vi "Cache.FindToExport.vi"(7 "Idx":i32, 8 "error in (no error)":errorcluster, 11 "Data in":T7) -> (0 "error out":errorcluster, 1 "ProductComponent":T1[](array[typedef]), 2 "Results":T2[](array[typedef]), 3 "Data out":T7)   [LabVIEW 2016]
uses:
  Cache.Data.ctl
  Cache.Data.Status.ctl
  Cache.Data.Sets.ctl
  Cache.TestSteps.Fglb.ResultData.ctl
  Database/ProdaNG/Controls/ProdaNG.ProcessResult.ctl
  Database/ProdaNG/Controls/ProdaNG.ProcessStepResult.ctl
  Database/ProdaNG/Controls/ProdaNG.TestStepResult.ctl
  Database/ProdaNG/Controls/ProdaNG.TestValueResult.ctl
  Database/ProdaNG/Controls/ProdaNG.ProductComponent.ctl
  Global/ApplicationGlobal.vi
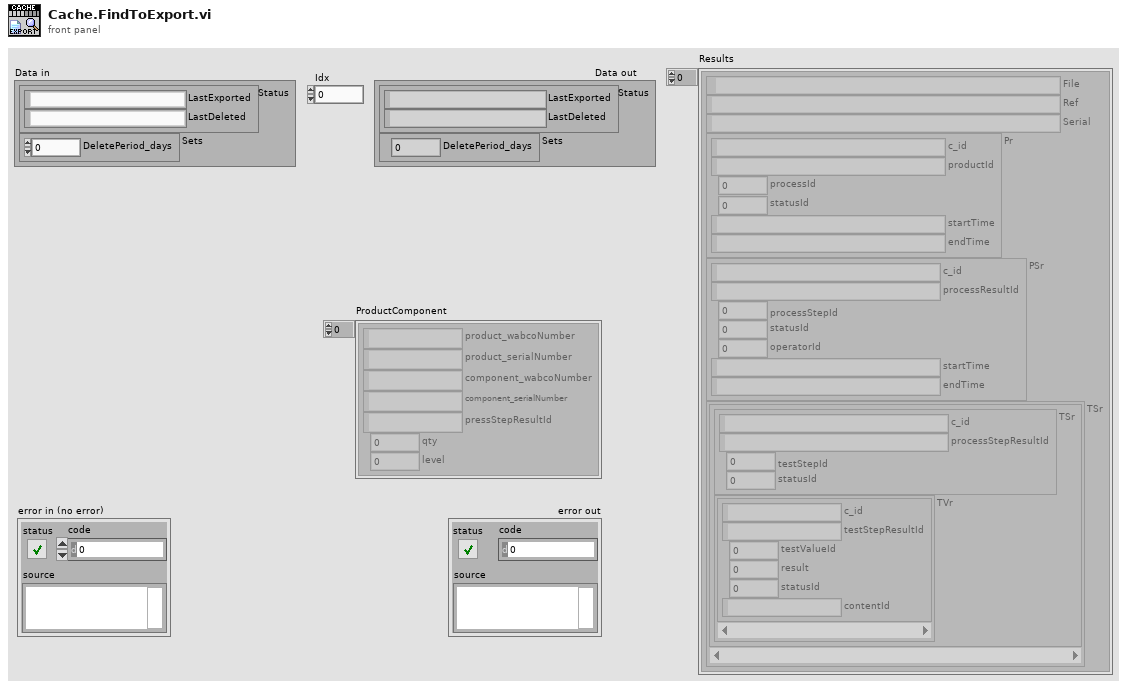
[diagram p1: front panel]
types:
  T1 = typedef "ProdaNG.ProductComponent.ctl" = cluster{"product_wabcoNumber":string, "product_serialNumber":string, "component_wabcoNumber":string, "component_serialNumber":string, "pressStepResultId":string, "qty":i32, "level":i32}
  T2 = typedef "Cache.TestSteps.Fglb.ResultData.ctl" = cluster{"File":path, "Ref":string, "Serial":string, "Pr":T3, "PSr":T4, "TSr":cluster{"TSr":T5, "TVr":T6[]}[]}
  T3 = typedef "ProdaNG.ProcessResult.ctl" = cluster{"c_id":string, "productId":string, "processId":i32, "statusId":i32, "startTime":string, "endTime":string}
  T4 = typedef "ProdaNG.ProcessStepResult.ctl" = cluster{"c_id":string, "processResultId":string, "processStepId":i32, "statusId":i32, "operatorId":i32, "startTime":string, "endTime":string}
  T5 = typedef "ProdaNG.TestStepResult.ctl" = cluster{"c_id":string, "processStepResultId":string, "testStepId":i32, "statusId":i32}
  T6 = typedef "ProdaNG.TestValueResult.ctl" = cluster{"c_id":string, "testStepResultId":string, "testValueId":i32, "result":dbl, "statusId":i32, "contentId":string}
  T7 = typedef "Cache.Data.ctl" = cluster{"Status":T8, "Sets":T9}
  T8 = typedef "Cache.Data.Status.ctl" = cluster{"LastExported":string, "LastDeleted":string}
  T9 = typedef "Cache.Data.Sets.ctl" = cluster{"DeletePeriod_days":dbl}
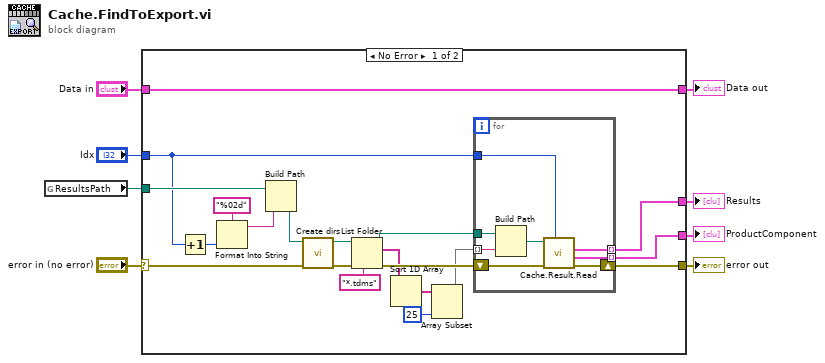
[diagram p0: block diagram]
diagram:
  n1 = global read "ApplicationGlobal.vi" "ResultsPath"() -> (w3:path)
  n2 = case shown="No Error" "error in (no error)" {
    selector: "error in (no error)" -> [w14 w37]
    tunnel: [w11 w37] -> w8
    tunnel: "Data in" -> [w27 w36]
    tunnel: [w27 w36] -> w5
    tunnel: [w9 _] -> w2
    tunnel: [w10 _] -> w1
    tunnel: "Idx" -> [w12 _]
    tunnel: w3 -> [w13 _]
    frame No Error {
      n3 = Increment(x=w12) -> (x+1=w21:i32)
      n4 = Format Into String(format string="%02d", w21) -> (resulting string=w23:string)  [unwired: 2 in, 1 out]
      n5 = Build Path(base path=w13, name or relative path=w23) -> (appended path=w15:path)
      n6 = call "Create dirs.vi"("error in (no error)"=w14, "deepest dir"=w15) -> ("error"=w16:errorcluster)  [unwired: 9 out]
      n7 = List Folder(path=w15, pattern="*.tdms", error in=w16) -> (path out=w25:path, filenames=w20:string[], error out=w26:errorcluster)  [unwired: 1 in, 1 out]
      n8 = Sort 1D Array(array=w20) -> (sorted array=w18:string[])
      n9 = Array Subset(array=w18, length=25) -> (w17:string[])  [unwired: 1 in]
      n10 = for {
        tunnel: w17 -> [w34] mode=indexing
        tunnel: w25 -> [w35]
        shift-right: [w32] -> w11
        shift-left: w26 -> [w33]
        tunnel: w12 -> [w30]
        tunnel: [w29] -> w10 mode=indexing
        tunnel: [w28] -> w9 mode=indexing
        # "through all files"
        n11 = Build Path(base path=w35, name or relative path=w34) -> (appended path=w31:path)
        n12 = call "Cache.Result.Read.vi"("Idx"=w30, "error in (no error)"=w33, "ResultsPath"=w31) -> ("error out"=w32:errorcluster, "ProductComponent"=w29:T1, "Result"=w28:T2)  [unwired: 6 in]
      }
    }
    frame Error {
    }
  }
  "error out" <- w8
  "Data out" <- w5
  "ProductComponent" <- w1
  "Results" <- w2
